vi "Query Capabilities (Power).vi"(0 "VISA resource name":refnum<visa-resource-name>, 5 "Absolute Maximums (T)":bool=TRUE, 11 "error in (no error)":errorcluster) -> (4 "VISA resource name out":refnum<visa-resource-name>, 6 "Power Capabilities":T1, 15 "error out":errorcluster)   [LabVIEW 2012, in "NH Research Regenerative Test Series.lvlib"]
doc: "Returns various Power capabilities of the module."
uses:
  <instrlib>/NH Research Regenerative Test Series/NH Research Regenerative Test Series.lvlib
  <instrlib>/NH Research Regenerative Test Series/Public/Utility/Power Capabilities.ctl
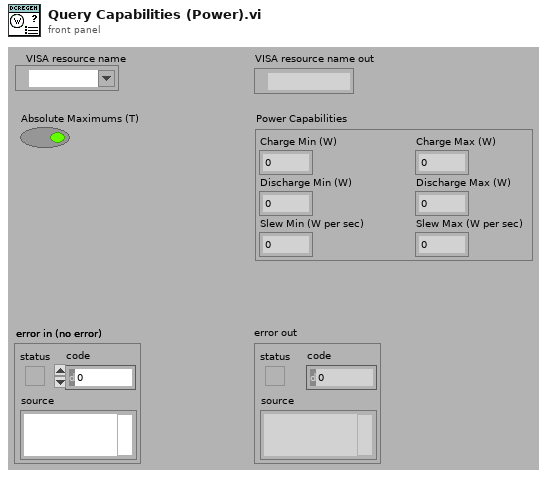
[diagram p1: front panel]
types:
  T1 = typedef "NH Research Regenerative Test Series.lvlib/Power Capabilities.ctl" = cluster{"Charge Min (W)":dbl, "Charge Max (W)":dbl, "Discharge Min (W)":dbl, "Discharge Max (W)":dbl, "Slew Min (W per sec)":dbl, "Slew Max (W per sec)":dbl}
  T2 = cluster{"[0]":dbl, "[1]":dbl, "[2]":dbl, "[3]":dbl, "[4]":dbl, "[5]":dbl}
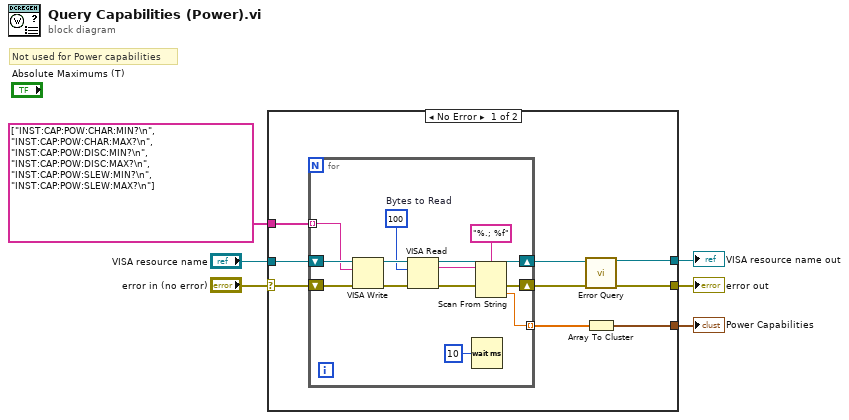
[diagram p0: block diagram]
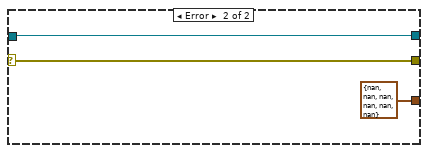
[diagram p2: hidden frame]
diagram:
  # "Not used for Power capabilities"
  n1 = case shown="No Error" "error in (no error)" {
    selector: "error in (no error)" -> [w14 w31]
    tunnel: [w9 w31] -> w5
    tunnel: [w15 w30] -> w3
    tunnel: "VISA resource name" -> [w13 w30]
    tunnel: string[] ["INST:CAP:POW:CHAR:MIN?\n", "INST:CAP:POW:CHAR:MAX?\n", "INST:CAP:POW:DISC:MIN?\n", "INST:CAP:POW:DISC:MAX?\n", "INST:CAP:POW:SLEW:MIN?\n", "INST:CAP:POW:SLEW:MAX?\n"] -> [w12 _]
    tunnel: [w8 T1 {"Charge Min (W)"=nan, "Charge Max (W)"=nan, "Discharge Min (W)"=nan, "Discharge Max (W)"=nan, "Slew Min (W per sec)"=nan, "Slew Max (W per sec)"=nan}] -> w1
    frame No Error {
      n2 = for {
        tunnel: w12 -> [w23] mode=indexing
        tunnel: [w19] -> w11 mode=indexing
        shift-right: [w18] -> w10
        shift-left: w14 -> [w25]
        shift-right: [w17] -> w7
        shift-left: w13 -> [w24]
        w26 = u32 100  # Bytes to Read
        n3 = VISA Write(VISA resource name=w24, write buffer=w23, error in (no error)=w25) -> (VISA resource name out=w27:refnum<visa-resource-name>, error out=w28:errorcluster)  [unwired: 1 out]
        n4 = VISA Read(VISA resource name=w27, byte count=w26, error in (no error)=w28) -> (VISA resource name out=w17:refnum<visa-resource-name>, read buffer=w20:string, error out=w21:errorcluster)  [unwired: 1 out]
        n5 = Wait (ms)(milliseconds to wait=u32 10) -> ()  [unwired: 1 out]
        n6 = Scan From String(format string="%.; %f", input string=w20, error in=w21) -> (error out=w18:errorcluster, output 1=w19:dbl)  [unwired: 2 in, 2 out]
      }
      n7 = call <instrlib>:"Error Query.vi"("VISA resource name"=w7, "error in (no error)"=w10) -> ("VISA resource name out"=w15:refnum<visa-resource-name>, "error out"=w9:errorcluster)  [unwired: 10 in, 2 out]
      n8 = Array To Cluster(array=w11) -> (cluster=w8:T2)
    }
    frame Error {
    }
  }
  "error out" <- w5
  "VISA resource name out" <- w3
  "Power Capabilities" <- w1
